vi "Target.vi"() -> ()   [LabVIEW 2017]
uses:
  shared/Kobuki Sensor Display.ctl
  controls/StatesEnum.ctl
  <vilib>/Platform/TimedLoop/XDataNode/timing_clust.ctl
  <vilib>/Platform/TimedLoop/XDataNode/nitl_modes.ctl
  <vilib>/Platform/TimedLoop/XDataNode/wakeup.ctl
  <vilib>/myRIO/Instrument Drivers/Onboard IO/UART/typedef/VISA Configuration.ctl
  shared/Sensors.ctl
  shared/Accelerometer.ctl
  Kobuki/KobukiSensors.ctl
  Kobuki/Kobuki Bumps and WheelDrops.ctl
  Kobuki/Kobuki Buttons.ctl
  <vilib>/myRIO/Common/Instrument Driver Framework/myRIO v1.0/UART/vis/myRIO v1.0 Close UART.vi
  <vilib>/myRIO/Common/Instrument Driver Framework/myRIO v1.0/myRIO v1.1 Open.vi
  <vilib>/Instr/_visa.llb/VISA Configure Serial Port (Instr).vi
  Global Light Sensor.vi
  <vilib>/myRIO/Common/Instrument Driver Framework/Utilities/vis/FPGA Ref Manager.vi
  <vilib>/myRIO/Common/Instrument Driver Framework/myRIO v1.0/myRIO v1.0 Reset FPGA.vi
  <vilib>/myRIO/Common/Instrument Driver Framework/myRIO v1.0/IRQ/vis/myRIO v1.0 IRQ Info FGV.vi
  <vilib>/myRIO/Common/Instrument Driver Framework/myRIO v1.0/IRQ/vis/myRIO v1.0 Timer IRQ Info FGV.vi
  <vilib>/myRIO/Common/Instrument Driver Framework/myRIO v1.0/IRQ/vis/myRIO v1.0 ISR Agent.vi
  <vilib>/Platform/TimedLoop/XDataNode/XDataNode.xnode
  <vilib>/myRIO/Express VI/Onboard IO/UART/UART Express VI.xnode
  <vilib>/myRIO/Instrument Drivers/Utilities/Utilities.lvlib
  <vilib>/Platform/TimedLoop/XDataNode/XDNodeRunTimeDep.lvlib
  <vilib>/myRIO/Instrument Drivers/Onboard IO/UART/UART.lvlib
panel:
  out "Green Light Sensed":bool
  out "Red Light Sensed":bool
  out "Iteration Duration":i64
  in  "stop 2":bool
  out "element":dbl
  out "element 2":dbl
  out "x .or. y?":bool
  in  "Pause":bool
  in  "Tab Control":T1(tab)
  out "Kobuki Sensors (graphical)":T2 {"Right Wheel (mm/s)" scale=-500.0..500.0; "Left Wheel (mm/s)" scale=-500.0..500.0}
  out "Charge Status":i8(ring) items=["DISCHARGING"=0, "DOCKING_CHARGED"=2, "DOCKING_CHARGING"=6, "ADAPTER_CHARGED"=18, "ADAPTER_CHARGING"=22]
  out "Kobuki Battery Voltage":dbl(knob)=12000.0 scale=12.0..16.4 scale format="%#.1f"
  out "CurrentState":T4
  out "Loop Duration":i64
  out "error out":errorcluster
  in  "stop":bool
  out "Target Running":bool
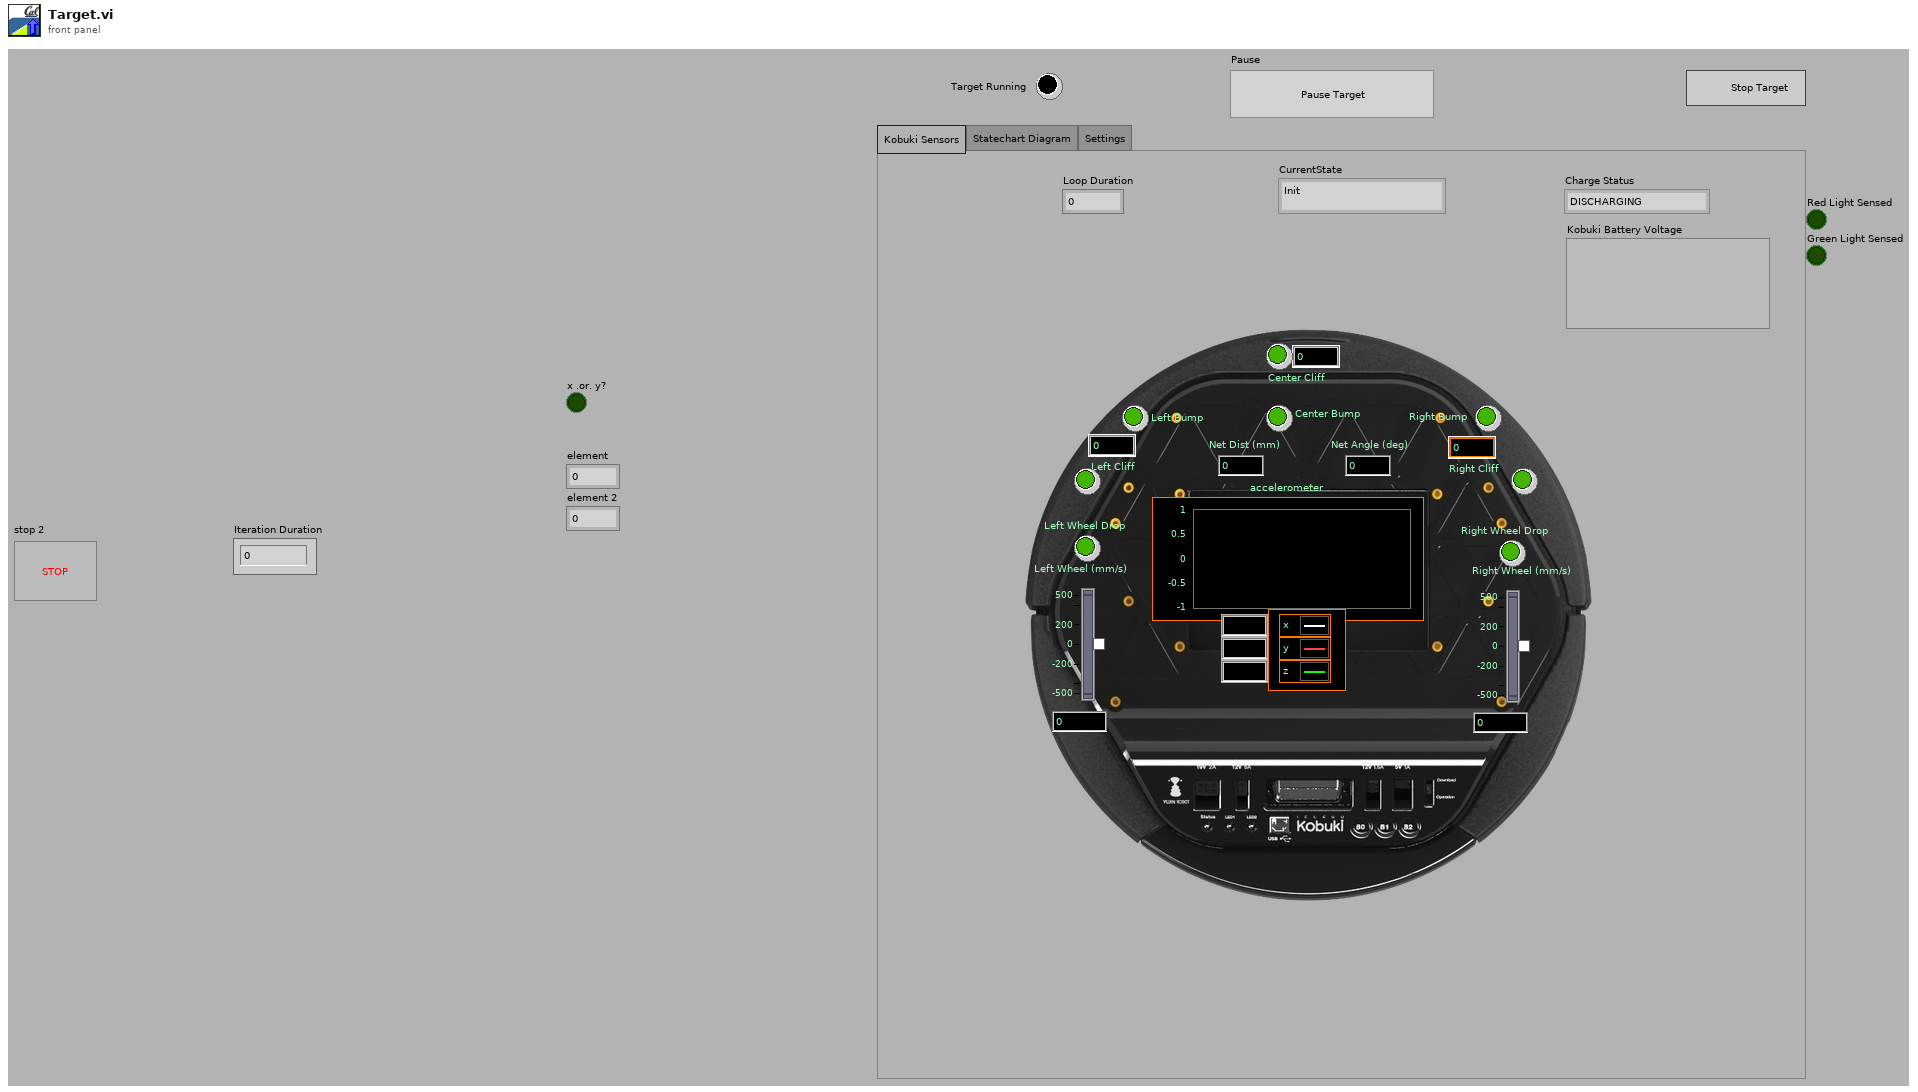
[diagram p1: front panel]
types:
  T1 = enum32{"Kobuki Sensors", "Statechart Diagram", "Settings"}
  T2 = typedef "Kobuki Sensor Display.ctl" = cluster{"Center Bump":bool, "Left Wheel Drop":bool, "Right Wheel Drop":bool, "Left Bump":bool, "Right Bump":bool, "Left Cliff":bool, "Center Cliff":bool, "Right Cliff":bool, "Net Dist (mm)":i32, "Net Angle (deg)":i32, "Left Cliff":u16, "Center Cliff":u16, "Right Cliff":u16, "  Left Wheel (mm/s)":i16, "Right Wheel (mm/s)":i16, "accelerometer":T3}
  T3 = typedef "Accelerometer.ctl" = cluster{"x axis (g)":dbl, "y axis (g)":dbl, "z axis (g)":dbl}
  T4 = typedef "StatesEnum.ctl" = enum16{"Init", "Center Cliff\n", "Pause", "Drive", "U.Turn", "L.Cliff", "R.Cliff", "Shut", "L.Bump", "R.Bump", "Red Light"}
  T5 = typedef "XDNodeRunTimeDep.lvlib/timing_clust.ctl" = cluster{"Expected End [f-1]":u64, "Actual End [f-1]":u64, "Finished Late? [f-1]":bool, "Expected End [i-1]":u64, "Actual End [i-1]":u64, "Finished Late? [i-1]":bool, "Expected Start [i]":u64, "Actual Start [i]":u64, "Expected Start [f]":u64, "Actual Start [f]":u64, "Source Name":string, "Structure Name":string, "Period":i64, "Deadline":i64, "Offset":i64, "Start":i64, "Priority":i32, "Timeout":i32, "Mode":T6, "Wakeup Reason":T7, "Error":errorcluster, "Source Type":string, "Secondary Source Type":string, "Global End Time":u64, "Global Start Time":u64, "Frame Duration":u64, "Iteration Duration":u64, "Assigned CPU":i32, "I/O Scan Engine Mode":u32}
  T6 = typedef "XDNodeRunTimeDep.lvlib/nitl_modes.ctl" = enum32{"No Change", "Process missed periods, maintain original phase", "Discard missed periods, maintain original phase", "Process missed periods, ignore original phase", "Discard missed periods, ignore original phase"}
  T7 = typedef "XDNodeRunTimeDep.lvlib/wakeup.ctl" = enum32{"Normal", "Aborted", "Asynchronous wakeup", "Timing source error", "Timed loop error", "Timeout"}
  T8 = typedef "IMAQ Image.ctl" = refnum<image>
  T9 = typedef "Sensors.ctl" = cluster{"net distance (mm)":i32, "net angle (deg)":i32, "accelerometer":T3, "Is Simulator?":bool, "Kobuki Sensors":T10, "Requested Left Wheel Velocity(mm/s)":i32, "Requested Right Wheel Velocity(mm/s)":i32, "Green Light Sensed":bool, "Red Light Sensed":bool}
  T10 = typedef "KobukiSensors.ctl" = cluster{"Bumps + Wheel Drops":T11, "Cliff Left":bool, "Cliff Center":bool, "Cliff Right":bool, "Cliff Left Signal":u16, "Cliff Center Signal":u16, "Cliff Right Signal":u16, "Buttons":T12, "Left Wheel Encoder (ticks)":u16, "Right Wheel Encoder (ticks) ":u16, "Left  Wheel PWM":i8, "Right Wheel PWM":i8, "Left Wheel OverCurrent":bool, "Right Wheel OverCurrent ":bool, "Right Wheel Current (x10mA)":i16, "Left  Wheel Current  (x10mA)":i16, "TimeStamp":u16, "Battery Voltage":dbl, "Angle( of 100deg)":i16, "Angle Rate( of 100 deg/sec)":i16, "Charger Source ":i8}
  T11 = typedef "Kobuki Bumps and WheelDrops.ctl" = cluster{"Wheeldrop Left":bool, "Wheeldrop Right":bool, "Bump Left":bool, "Bump Center":bool, "Bump Right":bool}
  T12 = typedef "Kobuki Buttons.ctl" = cluster{"B0":bool, "B1":bool, "B2":bool}
  T13 = typedef "Outputs.ctl" = cluster{"Left Wheel Speed (mm/s)":i16, "Right Wheel Speed (mm/s)":i16}
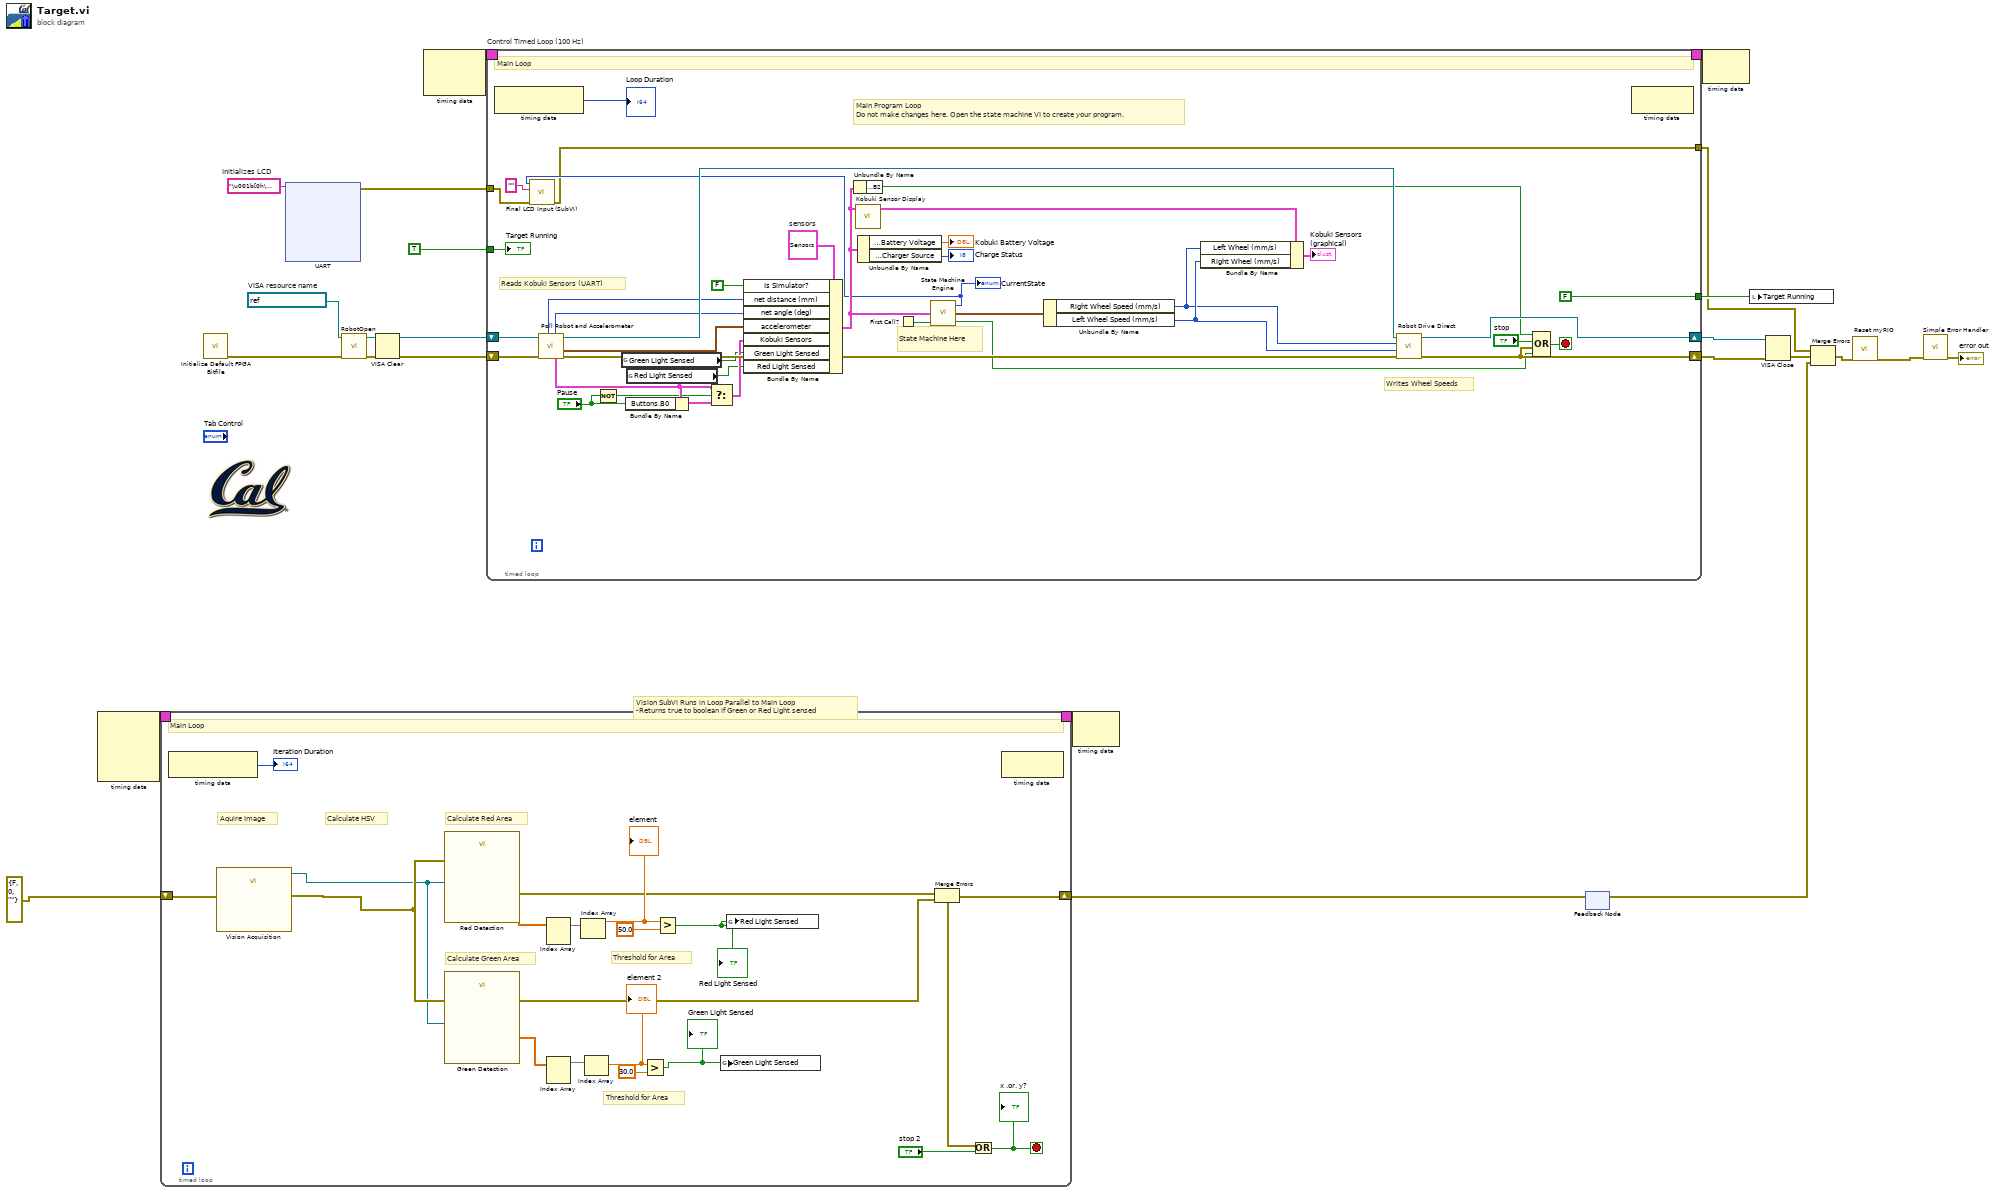
[diagram p0: block diagram]
diagram:
  w9 = "\u001b[0h\u001b[j"  # Initializes LCD
  w21 = refnum<visa-resource-name> "ASRL3::INSTR"  # VISA resource name
  # "Vision SubVI Runs in Loop Parallel to Main Loop\n-Returns true to boolean if Green or Red Light sensed"
  n1 = node-c288() -> (w5:T5)  [unwired: 4 in]
  n2 = timed-loop {
    shift-right: [w30] -> w2
    shift-left: errorcluster {"status"=FALSE, "code"=0, "source"=""} ("error in (no error)") -> [w43]
    timing: w5 -> [_]
    timing-out: [_] -> w4
    stop <- w29 stop-if-true
    # "Calculate Green Area"
    # "Calculate Red Area"
    # "Calculate HSV"
    # "Aquire Image"
    # "Threshold for Area"
    # "Threshold for Area"
    # "Main Loop"
    n3 = node-c288() -> (→"Iteration Duration":i64)  [unwired: 1 in]
    n4 = call "Vision Acquisition"("error in"=w43) -> ("Image Out"=w27:T8, "error out"=w28:errorcluster)  [unwired: 24 in, 1 out]
    n5 = call "Red Detection"("Image In"=w27, "error in"=w28) -> ("Particle Measurements (Pixels) (Particle Analysis 1)"=w39:dbl[][], "error out"=w32:errorcluster)  [unwired: 23 in, 1 out]
    n6 = call "Green Detection"("Image In"=w27, "error in"=w28) -> ("Particle Measurements (Pixels) (Particle Analysis 1)"=w36:dbl[][], "error out"=w31:errorcluster)  [unwired: 23 in, 1 out]
    n7 = Index Array(array=w39) -> (element=w34:dbl[])  [unwired: 2 in]
    n8 = Index Array(array=w36) -> (element=w38:dbl[])  [unwired: 2 in]
    n9 = Index Array(array=w34) -> (element=w42:dbl)  [unwired: 1 in]
    "element" <- w42
    n10 = Index Array(array=w38) -> (element=w37:dbl)  [unwired: 1 in]
    "element 2" <- w37
    n11 = Greater?(x=w37, y=30.0) -> (0:w25:bool)
    "Green Light Sensed" <- w25
    n12 = Greater?(x=w42, y=50.0) -> (0:w26:bool)
    "Red Light Sensed" <- w26
    n13 = global write "Global Light Sensor.vi" "Green Light Sensed"(w25) -> ()
    n14 = global write "Global Light Sensor.vi" "Red Light Sensed"(w26) -> ()
    n15 = Merge Errors(w32, w31) -> (w30:errorcluster)
    n16 = Or(x=w30, y="stop 2") -> (x .or. y?=w29:bool)
    "x .or. y?" <- w29
    n17 = node-c288() -> ()  [unwired: 1 in, 1 out]
  }
  n18 = call <vilib>:"Initialize Default FPGA Bitfile.vi"() -> ("error out"=w19:errorcluster)  [unwired: 11 in]
  n19 = xnode "UART"("Characters to Write"=w9) -> ("error out"=w10:errorcluster)  [unwired: 1 in, 1 out]
  n20 = call "RobotOpen.vi"("error in (no error)"=w19, "Robot Communication port name"=w21) -> ("error out"=w17:errorcluster, "Robot Communication port name out"=w24:refnum<visa-resource-name>)  [unwired: 8 in]
  n21 = VISA Clear(VISA resource name=w24, error in (no error)=w17) -> (VISA resource name out=w15:refnum<visa-resource-name>, error out=w16:errorcluster)
  n22 = node-c288() -> (w12:T5)  [unwired: 2 in]
  n23 = timed-loop "Control Timed Loop (100 Hz)" {
    shift-right: [w84] -> w13
    shift-left: w15 -> [w81]
    shift-right: [w69] -> w14
    shift-left: w16 -> [w80]
    tunnel: TRUE ("stop") -> [w75]
    tunnel: [FALSE ("stop")] -> w22
    timing: w12 -> [_]
    timing-out: [_] -> w11
    tunnel: w10 -> [w52]
    tunnel: [w49] -> w7
    stop <- w83 stop-if-true
    w70 = T9 {"net distance (mm)"=0, "net angle (deg)"=0, "accelerometer"={"x axis (g)"=0.0, "y axis (g)"=0.0, "z axis (g)"=0.0}, "Is Simulator?"=FALSE, "Kobuki Sensors"={"Bumps + Wheel Drops"={"Wheeldrop Left"=FALSE, "Wheeldrop Right"=FALSE, "Bump Left"=FALSE, "Bump Center"=FALSE, "Bump Right"=FALSE}, "Cliff Left"=FALSE, "Cliff Center"=FALSE, "Cliff Right"=FALSE, "Cliff Left Signal"=0, "Cliff Center Signal"=0, "Cliff Right Signal"=0, "Buttons"={"B0"=FALSE, "B1"=FALSE, "B2"=FALSE}, "Left Wheel Encoder (ticks)"=0, "Right Wheel Encoder (ticks) "=0, "Left  Wheel PWM"=0, "Right Wheel PWM"=0, "Left Wheel OverCurrent"=FALSE, "Right Wheel OverCurrent "=FALSE, "Right Wheel Current (x10mA)"=0, "Left  Wheel Current  (x10mA)"=0, "TimeStamp"=0, "Battery Voltage"=0.0, "Angle( of 100deg)"=0, "Angle Rate( of 100 deg/sec)"=0, "Charger Source "=0}, "Requested Left Wheel Velocity(mm/s)"=0, "Requested Right Wheel Velocity(mm/s)"=0, "Green Light Sensed"=FALSE, "Red Light Sensed"=FALSE}  # sensors
    # "Main Program Loop\nDo not make changes here. Open the state machine VI to create your program."
    # "Writes Wheel Speeds"
    # "Reads Kobuki Sensors (UART)"
    # "State Machine Here"
    # "Main Loop"
    n24 = node-c288() -> (→"Loop Duration":i64)  [unwired: 1 in]
    n25 = call "Poll Robot and Accelerometer.vi"("error in"=w80, "UART in"=w81) -> ("error out"=w79:errorcluster, "Acceleration (g)"=w72:T3, "UART out"=w78:refnum<visa-resource-name>, "Kobuki Sensors  out"=w56:T10, "net angle (deg)"=w76:i32, "net distance (mm)"=w77:i32)  [unwired: 4 in]
    n26 = Not(x="Pause") -> (.not. x?=w53:bool)
    n27 = global read "Global Light Sensor.vi" "Green Light Sensed"() -> (w48:bool)
    n28 = Bundle By Name(cluster=w56, "Buttons.B0"="Pause") -> (w57:T10)
    n29 = global read "Global Light Sensor.vi" "Red Light Sensed"() -> (w47:bool)
    n30 = Select(t=w56, s=w53, f=w57) -> (s? t:f=w55:T10)
    n31 = Bundle By Name(cluster=w70, "Is Simulator?"=FALSE, "net distance (mm)"=w77, "net angle (deg)"=w76, "accelerometer"=w72, "Kobuki Sensors"=w55, "Green Light Sensed"=w48, "Red Light Sensed"=w47) -> (w62:T9)
    n32 = Unbundle By Name(w62) -> ("Kobuki Sensors.Buttons.B2"=w73:bool)
    n33 = call "Kobuki Sensor Display.vi"("sensors"=w62) -> ("Kobuki Sensors Display"=w59:T2)  [unwired: 4 in]
    n34 = Unbundle By Name(w62) -> ("Kobuki Sensors.Battery Voltage"=→"Kobuki Battery Voltage":dbl, "Kobuki Sensors.Charger Source"=→"Charge Status":i8)
    n35 = First Call?() -> (First Call?: T/F=w64:bool)
    n36 = call "State Machine Engine.vi"("Init?"=w64, "Inputs"=w62) -> ("Terminated?"=w63:bool, "Outputs"=w67:T13, "state out"=w50:T4)  [unwired: 1 in]
    "CurrentState" <- w50
    n37 = call "Final LCD Input (SubVI).vi"("error in (no error)"=w52, "String Input"="", "state input"=w50) -> ("error out"=w49:errorcluster)  [unwired: 8 in]
    n38 = Unbundle By Name(w67) -> ("Right Wheel Speed (mm/s)"=w60:i16, "Left Wheel Speed (mm/s)"=w61:i16)
    n39 = Bundle By Name(cluster=w59, "Left Wheel (mm/s)"=w60, "Right Wheel (mm/s)"=w61) -> (→"Kobuki Sensors (graphical)":T2)
    n40 = call "Robot Drive Direct.vi"("error in"=w79, "Left Wheel Velocity (mm/s)"=w61, "Right Wheel Velocity (mm/s)"=w60, "UART port in"=w78) -> ("error out"=w69:errorcluster, "UART port out"=w84:refnum<visa-resource-name>)  [unwired: 6 in]
    n41 = Compound Arithmetic op=OR(w73, "stop", w69, w63) -> (w83:bool)
    n42 = node-c288() -> ()  [unwired: 1 in, 1 out]
    "Target Running" <- w75
  }
  n43 = node-c288(w4) -> ()  [unwired: 1 out]
  n44 = feedback-in #1(w2) -> ()
  n45 = feedback #1() -> (w1:errorcluster)  [unwired: 1 in]
  n46 = node-c288(w11) -> ()  [unwired: 1 out]
  n47 = local write "Target Running"(w22) -> ()
  n48 = VISA Close(VISA resource name=w13, error in (no error)=w14) -> (error out=w8:errorcluster)
  n49 = Merge Errors(w7, w8, w1) -> (w6:errorcluster)
  n50 = call <vilib>:"Reset myRIO.vi"("error in (no error)"=w6) -> ("error out"=w20:errorcluster)  [unwired: 10 in]
  n51 = call <vilib>:"Simple Error Handler.vi"("error in (no error)"=w20) -> ("error out"=→"error out":errorcluster)  [unwired: 4 in, 4 out]
